vi "Accelerator button.vi"() -> ()   [LabVIEW 2011]
panel:
  out "Meter 2":dbl(knob) scale=0.0..10.0
  in  "stop":bool
  in  "Accelerate":bool
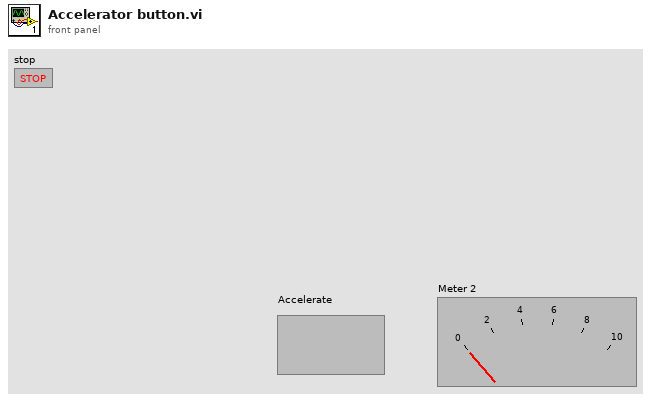
[diagram p1: front panel]
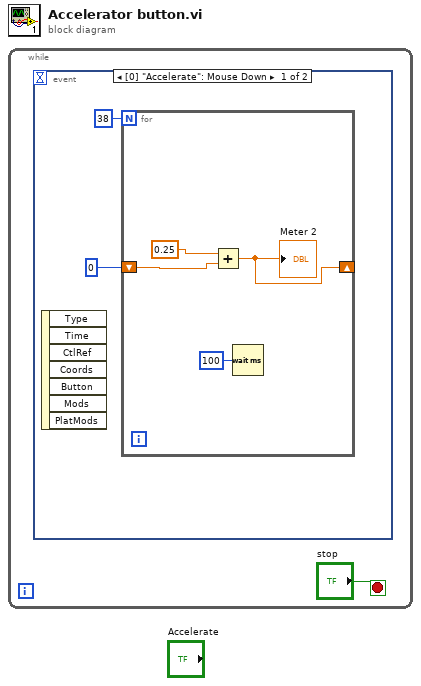
[diagram p0: block diagram]
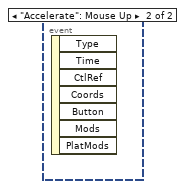
[diagram p2: hidden frame]
diagram:
  n1 = while {
    stop <- "stop" stop-if-true
    n2 = event shown="[0] \"Accelerate\": Mouse Down" {
      selector: _ -> [_ _]
      dyn-events: _ -> [_ _]
      timeout: _ -> [_ _]
      event "Accelerate": Mouse Down {
        n3 = event-data() -> ()  [unwired: 1 in, 7 out]
        n4 = for {
          N: 38 -> [_]
          shift-right: [w4] -> _
          shift-left: 0 ("y") -> [w6]
          n5 = Add(x=0.25, y=w6) -> (x+y=w4:dbl)
          "Meter 2" <- w4
          n6 = Wait (ms)(milliseconds to wait=u32 100) -> ()  [unwired: 1 out]
        }
      }
      event "Accelerate": Mouse Up {
        n7 = event-data() -> ()  [unwired: 1 in, 7 out]
      }
    }
  }
